vi "ModifyOrder.vi"(11 "buffer.in":u64[](array[numeric])=[0, 0, 0, 0, 0, 0, 0, 0, 0]) -> (3 "OrderBook.Command":T1)   [LabVIEW 2020]
doc: "Cboe PITCH Modify Order (0x27 long, 0x28 short) -> orderbook.command: type ModifyOrder, orderId, new quantity, new price, nanoseconds, Edit. Short price keeps 2 implied decimals (as AddOrder short does)."
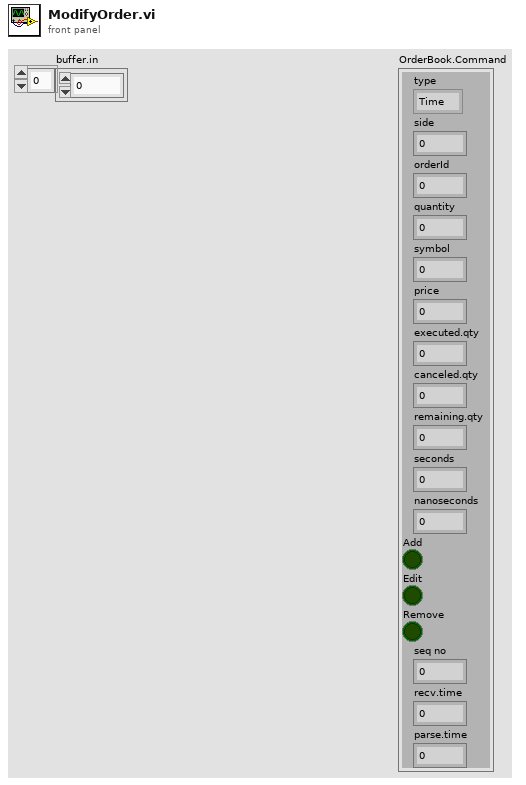
[diagram p1: front panel]
types:
  T1 = cluster{"type":enum8{"Time", "AddOrder", "OrderExecuted", "OrderExecutedAtPrice", "ReduceSize", "ModifyOrder", "DeleteOrder", "Get.Everything", "Get.All.Orders", "Get.Top"}, "side":u8, "orderId ":u64, "quantity":u32, "symbol":u64, "price":u64, "executed.qty":u32, "canceled.qty":u32, "remaining.qty":u32, "seconds":u64, "nanoseconds":u64, "Add":bool, "Edit":bool, "Remove":bool, "seq no":u32, "recv.time":u64, "parse.time":u64}
  T2 = enum8{"Time", "AddOrder", "OrderExecuted", "OrderExecutedAtPrice", "ReduceSize", "ModifyOrder", "DeleteOrder", "Get.Everything", "Get.All.Orders", "Get.Top"}
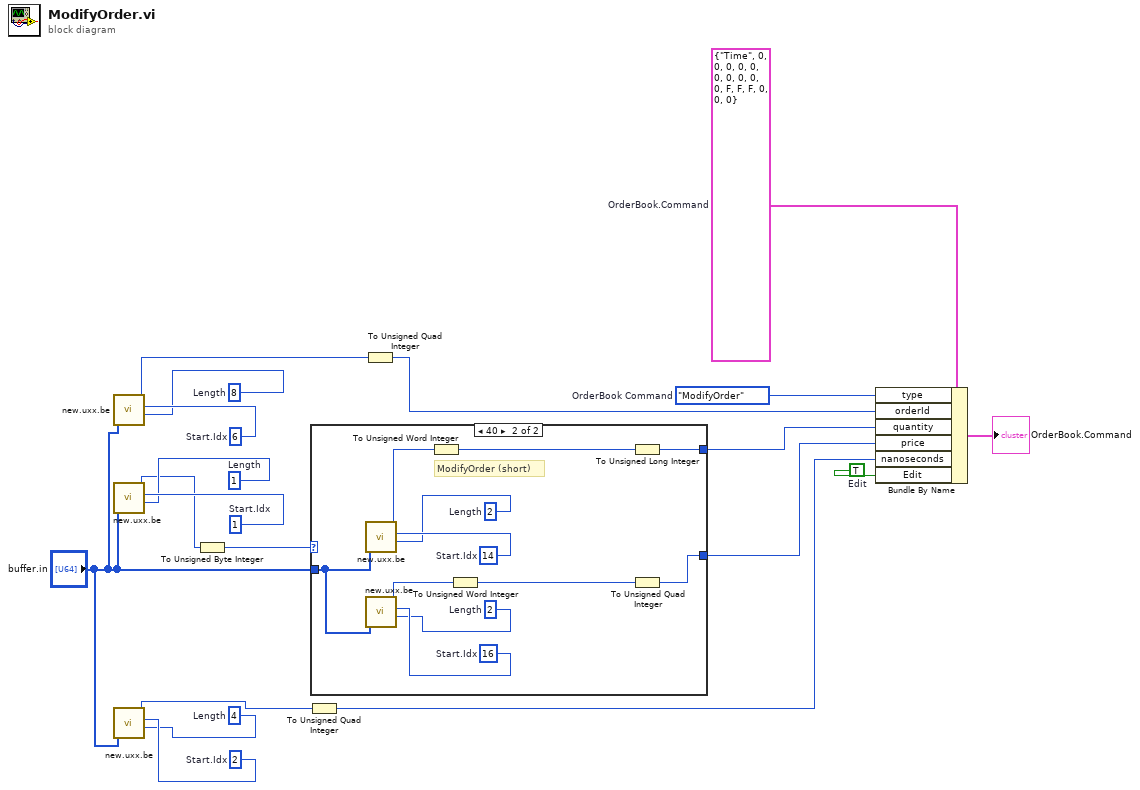
[diagram p0: block diagram]
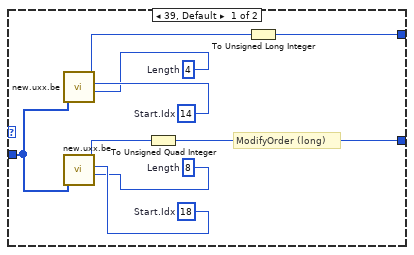
[diagram p2: hidden frame]
diagram:
  w12 = u8 8  # Length
  w13 = u8 6  # Start.Idx
  w15 = u8 4  # Length
  w16 = u8 2  # Start.Idx
  w18 = u8 1  # Length
  w19 = u8 1  # Start.Idx
  w3 = TRUE  # Edit
  w8 = T2."ModifyOrder"  # OrderBook Command
  w2 = T1 {"type"=enum."Time", "side"=0, "orderId "=0, "quantity"=0, "symbol"=0, "price"=0, "executed.qty"=0, "canceled.qty"=0, "remaining.qty"=0, "seconds"=0, "nanoseconds"=0, "Add"=FALSE, "Edit"=FALSE, "Remove"=FALSE, "seq no"=0, "recv.time"=0, "parse.time"=0}  # OrderBook.Command
  n1 = call "new.uxx.be.vi"("buffer (U64)"="buffer.in", "Start.Idx"=w13, "Length"=w12) -> ("Out.Value U64"=w11:u64)  [unwired: 7 in]
  n2 = call "new.uxx.be.vi"("buffer (U64)"="buffer.in", "Start.Idx"=w19, "Length"=w18) -> ("Out.Value U64"=w17:u64)  [unwired: 7 in]
  n3 = call "new.uxx.be.vi"("buffer (U64)"="buffer.in", "Start.Idx"=w16, "Length"=w15) -> ("Out.Value U64"=w14:u64)  [unwired: 7 in]
  n4 = To Unsigned Byte Integer(number=w17) -> (unsigned 8bit integer=w9:u8)
  n5 = To Unsigned Quad Integer(1:w14) -> (0:w4:u64)
  n6 = case shown="40" w9 {
    tunnel: "buffer.in" -> [w25 w35]
    tunnel: [w21 w30] -> w6
    tunnel: [w20 w29] -> w5
    frame 39, Default {
      w23 = u8 8  # Length
      w24 = u8 18  # Start.Idx
      w27 = u8 4  # Length
      w28 = u8 14  # Start.Idx
      # "ModifyOrder (long)"
      n7 = call "new.uxx.be.vi"("buffer (U64)"=w25, "Start.Idx"=w28, "Length"=w27) -> ("Out.Value U64"=w26:u64)  [unwired: 7 in]
      n8 = call "new.uxx.be.vi"("buffer (U64)"=w25, "Start.Idx"=w24, "Length"=w23) -> ("Out.Value U64"=w22:u64)  [unwired: 7 in]
      n9 = To Unsigned Quad Integer(1:w22) -> (0:w20:u64)
      n10 = To Unsigned Long Integer(number=w26) -> (unsigned 32bit integer=w21:u32)
    }
    frame 40 {
      w33 = u8 2  # Length
      w34 = u8 16  # Start.Idx
      w38 = u8 2  # Length
      w39 = u8 14  # Start.Idx
      # "ModifyOrder (short)"
      n11 = call "new.uxx.be.vi"("buffer (U64)"=w35, "Start.Idx"=w39, "Length"=w38) -> ("Out.Value U64"=w37:u64)  [unwired: 7 in]
      n12 = call "new.uxx.be.vi"("buffer (U64)"=w35, "Start.Idx"=w34, "Length"=w33) -> ("Out.Value U64"=w32:u64)  [unwired: 7 in]
      n13 = To Unsigned Word Integer(number=w37) -> (unsigned 16bit integer=w36:u16)
      n14 = To Unsigned Word Integer(number=w32) -> (unsigned 16bit integer=w31:u16)
      n15 = To Unsigned Long Integer(number=w36) -> (unsigned 32bit integer=w30:u32)
      n16 = To Unsigned Quad Integer(1:w31) -> (0:w29:u64)
    }
  }
  n17 = To Unsigned Quad Integer(1:w11) -> (0:w7:u64)
  n18 = Bundle By Name(cluster=w2, "type"=w8, "orderId"=w7, "quantity"=w6, "price"=w5, "nanoseconds"=w4, "Edit"=w3) -> (→"OrderBook.Command":T1)
